vi "LidarTest.vi"() -> ()   [LabVIEW 2012]
uses:
  <instrlib>/Hokuyo URG Series/Public/Initialize-Standard.vi
  <instrlib>/Hokuyo URG Series/Hokuyo URG Series.lvlib
panel:
  out "Waveform Chart":i32(graph)
  out "size(s)":i32=961
  out "Direction":dbl[](array[numeric])
  out "Magnitude":dbl[](array[numeric])
  out "XY Graph":cluster{"X":dbl, "Y":dbl}[](graph)
  in  "polar attributes (hidden)":T1={"maximum"=30000.0, "minimum"=0.0, "clip to min"=FALSE, "log?(F)"=TRUE, "grid color"=6710886, "plot color"=65280, "fmt and prec"={"format"=enum."Decimal", "precision"=0}, "visible section"=8} {"minimum" format="%0.2f"; "maximum" format="%0.2f"}
  in  "Protocol":u32(ring)=2 items=["Convert to Latest", "SCIP 1.1", "SCIP 2.0"]
  in  "ID Query?":bool=TRUE
  in  "Checksum":bool
  in  "VISA resource name":refnum<visa-resource-name>="TCPIP::192.168.0.10::10940::SOCKET"
  in  "Stop":bool
  out "Data Aquired":picture
  in  "Grid Color":u32(colorbox)=16777222
  in  "Plot Color":u32(colorbox)=6618880
  in  "Max (m)":dbl=4.1
  in  "End Point":dbl=120.0
  in  "Start Point":dbl=-120.0
  in  "Cluster Count":dbl=1.0
  in  "Encoding Width":u16(ring)=3 items=["2 Byte"=2, "3 Byte"=3]
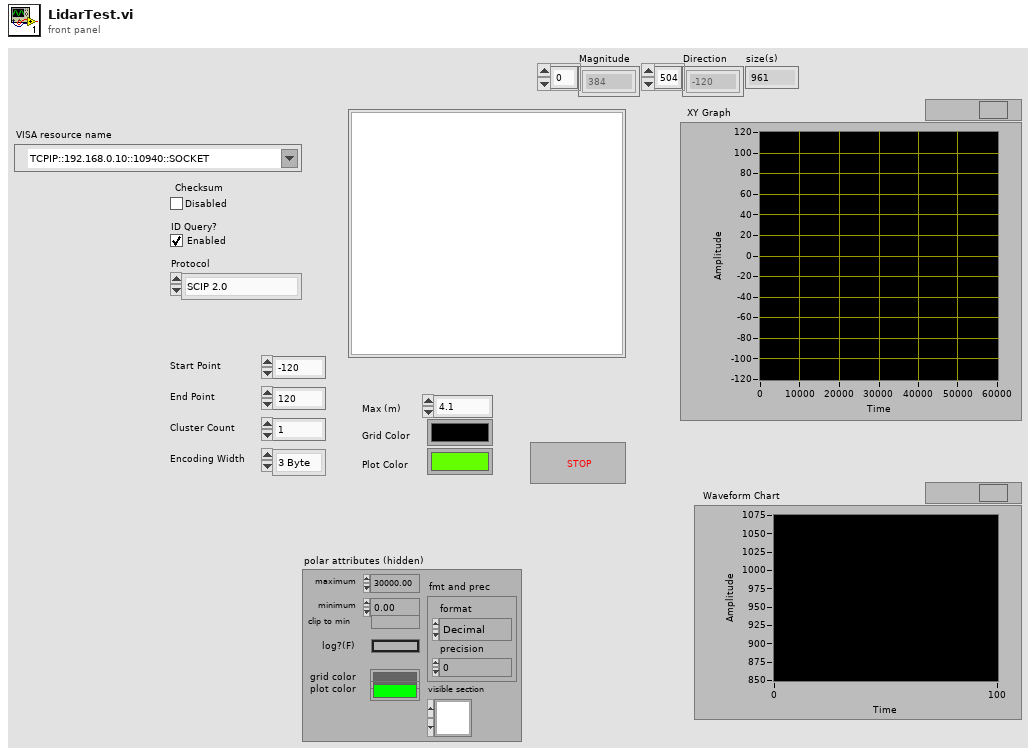
[diagram p1: front panel]
types:
  T1 = cluster{"maximum":dbl, "minimum":dbl, "clip to min":bool, "log?(F)":bool, "grid color":u32, "plot color":u32, "fmt and prec":cluster{"format":enum8{"Decimal", "Scientific", "Engineering", "Binary", "Octal", "Hex"}, "precision":u8}, "visible section":u16}
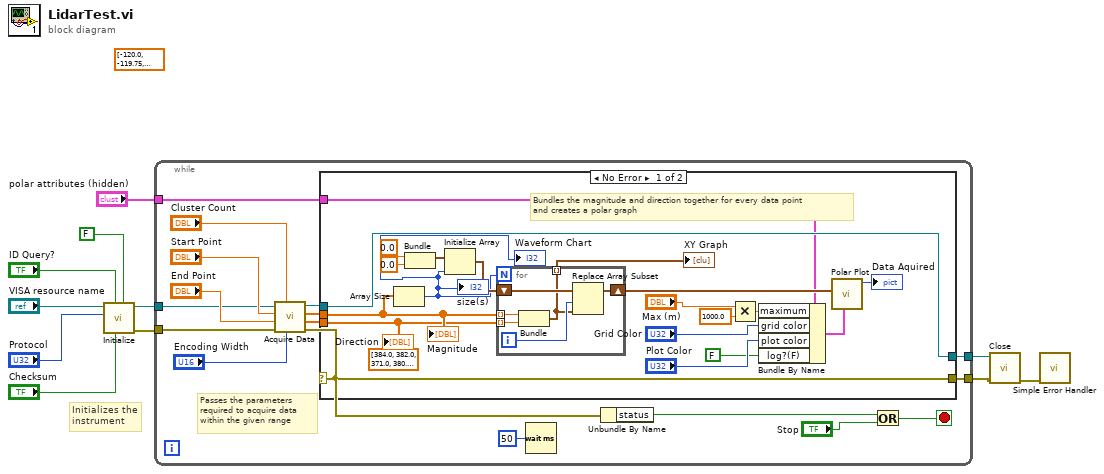
[diagram p0: block diagram]
diagram:
  (unwired) dbl[] [-120.0, -119.75, -119.5, -119.25, -119.0, -118.75, -118.5, -118.25, -118.0, -117.75, -117.5, -117.25, -117.0, -116.75, -116.5, -116.25, -116.0, -115.75, -115.5, -115.25, -115.0, -114.75, -114.5, -114.25, -114.0, -113.75, -113.5, -113.25, -113.0, -112.75, -112.5, -112.25, -112.0, -111.75, -111.5, -111.25, -111.0, -110.75, -110.5, -110.25, -110.0, -109.75, -109.5, -109.25, -109.0, -108.75, -108.5, -108.25, -108.0, -107.75, -107.5, -107.25, -107.0, -106.75, -106.5, -106.25, -106.0, -105.75, -105.5, -105.25, -105.0, -104.75, -104.5, -104.25, -104.0, -103.75, -103.5, -103.25, -103.0, -102.75, -102.5, -102.25, -102.0, -101.75, -101.5, -101.25, -101.0, -100.75, -100.5, -100.25, -100.0, -99.75, -99.5, -99.25, -99.0, -98.75, -98.5, -98.25, -98.0, -97.75, -97.5, -97.25, -97.0, -96.75, -96.5, -96.25, -96.0, -95.75, -95.5, -95.25, -95.0, -94.75, -94.5, -94.25, -94.0, -93.75, -93.5, -93.25, -93.0, -92.75, -92.5, -92.25, -92.0, -91.75, -91.5, -91.25, -91.0, -90.75, -90.5, -90.25, -90.0, -89.75, -89.5, -89.25, -89.0, -88.75, -88.5, -88.25, -88.0, -87.75, -87.5, -87.25, -87.0, -86.75, -86.5, -86.25, -86.0, -85.75, -85.5, -85.25, -85.0, -84.75, -84.5, -84.25, -84.0, -83.75, -83.5, -83.25, -83.0, -82.75, -82.5, -82.25, -82.0, -81.75, -81.5, -81.25, -81.0, -80.75, -80.5, -80.25, -80.0, -79.75, -79.5, -79.25, -79.0, -78.75, -78.5, -78.25, -78.0, -77.75, -77.5, -77.25, -77.0, -76.75, -76.5, -76.25, -76.0, -75.75, -75.5, -75.25, -75.0, -74.75, -74.5, -74.25, -74.0, -73.75, -73.5, -73.25, -73.0, -72.75, -72.5, -72.25, -72.0, -71.75, -71.5, -71.25, -71.0, -70.75, -70.5, -70.25, -70.0, -69.75, -69.5, -69.25, -69.0, -68.75, -68.5, -68.25, -68.0, -67.75, -67.5, -67.25, -67.0, -66.75, -66.5, -66.25, -66.0, -65.75, -65.5, -65.25, -65.0, -64.75, -64.5, -64.25, -64.0, -63.75, -63.5, -63.25, -63.0, -62.75, -62.5, -62.25, -62.0, -61.75, -61.5, -61.25, -61.0, -60.75, -60.5, -60.25, -60.0, -59.75, -59.5, -59.25, -59.0, -58.75, -58.5, -58.25, -58.0, -57.75, -57.5, -57.25, -57.0, -56.75, -56.5, -56.25, -56.0, -55.75, -55.5, -55.25, -55.0, -54.75, -54.5, -54.25, -54.0, -53.75, -53.5, -53.25, -53.0, -52.75, -52.5, -52.25, -52.0, -51.75, -51.5, -51.25, -51.0, -50.75, -50.5, -50.25, -50.0, -49.75, -49.5, -49.25, -49.0, -48.75, -48.5, -48.25, -48.0, -47.75, -47.5, -47.25, -47.0, -46.75, -46.5, -46.25, -46.0, -45.75, -45.5, -45.25, -45.0, -44.75, -44.5, -44.25, -44.0, -43.75, -43.5, -43.25, -43.0, -42.75, -42.5, -42.25, -42.0, -41.75, -41.5, -41.25, -41.0, -40.75, -40.5, -40.25, -40.0, -39.75, -39.5, -39.25, -39.0, -38.75, -38.5, -38.25, -38.0, -37.75, -37.5, -37.25, -37.0, -36.75, -36.5, -36.25, -36.0, -35.75, -35.5, -35.25, -35.0, -34.75, -34.5, -34.25, -34.0, -33.75, -33.5, -33.25, -33.0, -32.75, -32.5, -32.25, -32.0, -31.75, -31.5, -31.25, -31.0, -30.75, -30.5, -30.25, -30.0, -29.75, -29.5, -29.25, -29.0, -28.75, -28.5, -28.25, -28.0, -27.75, -27.5, -27.25, -27.0, -26.75, -26.5, -26.25, -26.0, -25.75, -25.5, -25.25, -25.0, -24.75, -24.5, -24.25, -24.0, -23.75, -23.5, -23.25, -23.0, -22.75, -22.5, -22.25, -22.0, -21.75, -21.5, -21.25, -21.0, -20.75, -20.5, -20.25, -20.0, -19.75, -19.5, -19.25, -19.0, -18.75, -18.5, -18.25, -18.0, -17.75, -17.5, -17.25, -17.0, -16.75, -16.5, -16.25, -16.0, -15.75, -15.5, -15.25, -15.0, -14.75, -14.5, -14.25, -14.0, -13.75, -13.5, -13.25, -13.0, -12.75, -12.5, -12.25, -12.0, -11.75, -11.5, -11.25, -11.0, -10.75, -10.5, -10.25, -10.0, -9.75, -9.5, -9.25, -9.0, -8.75, -8.5, -8.25, -8.0, -7.75, -7.5, -7.25, -7.0, -6.75, -6.5, -6.25, -6.0, -5.75, -5.5, -5.25, -5.0, -4.75, -4.5, -4.25, -4.0, -3.75, -3.5, -3.25, -3.0, -2.75, -2.5, -2.25, -2.0, -1.75, -1.5, -1.25, -1.0, -0.75, -0.5, -0.25, 0.0, 0.25, 0.5, 0.75, 1.0, 1.25, 1.5, 1.75, 2.0, 2.25, 2.5, 2.75, 3.0, 3.25, 3.5, 3.75, 4.0, 4.25, 4.5, 4.75, 5.0, 5.25, 5.5, 5.75, 6.0, 6.25, 6.5, 6.75, 7.0, 7.25, 7.5, 7.75, 8.0, 8.25, 8.5, 8.75, 9.0, 9.25, 9.5, 9.75, 10.0, 10.25, 10.5, 10.75, 11.0, 11.25, 11.5, 11.75, 12.0, 12.25, 12.5, 12.75, 13.0, 13.25, 13.5, 13.75, 14.0, 14.25, 14.5, 14.75, 15.0, 15.25, 15.5, 15.75, 16.0, 16.25, 16.5, 16.75, 17.0, 17.25, 17.5, 17.75, 18.0, 18.25, 18.5, 18.75, 19.0, 19.25, 19.5, 19.75, 20.0, 20.25, 20.5, 20.75, 21.0, 21.25, 21.5, 21.75, 22.0, 22.25, 22.5, 22.75, 23.0, 23.25, 23.5, 23.75, 24.0, 24.25, 24.5, 24.75, 25.0, 25.25, 25.5, 25.75, 26.0, 26.25, 26.5, 26.75, 27.0, 27.25, 27.5, 27.75, 28.0, 28.25, 28.5, 28.75, 29.0, 29.25, 29.5, 29.75, 30.0, 30.25, 30.5, 30.75, 31.0, 31.25, 31.5, 31.75, 32.0, 32.25, 32.5, 32.75, 33.0, 33.25, 33.5, 33.75, 34.0, 34.25, 34.5, 34.75, 35.0, 35.25, 35.5, 35.75, 36.0, 36.25, 36.5, 36.75, 37.0, 37.25, 37.5, 37.75, 38.0, 38.25, 38.5, 38.75, 39.0, 39.25, 39.5, 39.75, 40.0, 40.25, 40.5, 40.75, 41.0, 41.25, 41.5, 41.75, 42.0, 42.25, 42.5, 42.75, 43.0, 43.25, 43.5, 43.75, 44.0, 44.25, 44.5, 44.75, 45.0, 45.25, 45.5, 45.75, 46.0, 46.25, 46.5, 46.75, 47.0, 47.25, 47.5, 47.75, 48.0, 48.25, 48.5, 48.75, 49.0, 49.25, 49.5, 49.75, 50.0, 50.25, 50.5, 50.75, 51.0, 51.25, 51.5, 51.75, 52.0, 52.25, 52.5, 52.75, 53.0, 53.25, 53.5, 53.75, 54.0, 54.25, 54.5, 54.75, 55.0, 55.25, 55.5, 55.75, 56.0, 56.25, 56.5, 56.75, 57.0, 57.25, 57.5, 57.75, 58.0, 58.25, 58.5, 58.75, 59.0, 59.25, 59.5, 59.75, 60.0, 60.25, 60.5, 60.75, 61.0, 61.25, 61.5, 61.75, 62.0, 62.25, 62.5, 62.75, 63.0, 63.25, 63.5, 63.75, 64.0, 64.25, 64.5, 64.75, 65.0, 65.25, 65.5, 65.75, 66.0, 66.25, 66.5, 66.75, 67.0, 67.25, 67.5, 67.75, 68.0, 68.25, 68.5, 68.75, 69.0, 69.25, 69.5, 69.75, 70.0, 70.25, 70.5, 70.75, 71.0, 71.25, 71.5, 71.75, 72.0, 72.25, 72.5, 72.75, 73.0, 73.25, 73.5, 73.75, 74.0, 74.25, 74.5, 74.75, 75.0, 75.25, 75.5, 75.75, 76.0, 76.25, 76.5, 76.75, 77.0, 77.25, 77.5, 77.75, 78.0, 78.25, 78.5, 78.75, 79.0, 79.25, 79.5, 79.75, 80.0, 80.25, 80.5, 80.75, 81.0, 81.25, 81.5, 81.75, 82.0, 82.25, 82.5, 82.75, 83.0, 83.25, 83.5, 83.75, 84.0, 84.25, 84.5, 84.75, 85.0, 85.25, 85.5, 85.75, 86.0, 86.25, 86.5, 86.75, 87.0, 87.25, 87.5, 87.75, 88.0, 88.25, 88.5, 88.75, 89.0, 89.25, 89.5, 89.75, 90.0, 90.25, 90.5, 90.75, 91.0, 91.25, 91.5, 91.75, 92.0, 92.25, 92.5, 92.75, 93.0, 93.25, 93.5, 93.75, 94.0, 94.25, 94.5, 94.75, 95.0, 95.25, 95.5, 95.75, 96.0, 96.25, 96.5, 96.75, 97.0, 97.25, 97.5, 97.75, 98.0, 98.25, 98.5, 98.75, 99.0, 99.25, 99.5, 99.75, 100.0, 100.25, 100.5, 100.75, 101.0, 101.25, 101.5, 101.75, 102.0, 102.25, 102.5, 102.75, 103.0, 103.25, 103.5, 103.75, 104.0, 104.25, 104.5, 104.75, 105.0, 105.25, 105.5, 105.75, 106.0, 106.25, 106.5, 106.75, 107.0, 107.25, 107.5, 107.75, 108.0, 108.25, 108.5, 108.75, 109.0, 109.25, 109.5, 109.75, 110.0, 110.25, 110.5, 110.75, 111.0, 111.25, 111.5, 111.75, 112.0, 112.25, 112.5, 112.75, 113.0, 113.25, 113.5, 113.75, 114.0, 114.25, 114.5, 114.75, 115.0, 115.25, 115.5, 115.75, 116.0, 116.25, 116.5, 116.75, 117.0, 117.25, 117.5, 117.75, 118.0, 118.25, 118.5, 118.75, 119.0, 119.25, 119.5, 119.75, 120.0] ("Direction")
  # "Initializes the instrument"
  n1 = call-poly <instrlib>:"Initialize.vi"("Reset? (F: No)"=FALSE ("Reset Instrument (Disabled)"), "Checksum (Disabled)"="Checksum", "ID Query? (Enabled)"="ID Query?", "Protocol (2: SCIP 2.0)"="Protocol", "VISA resource name"="VISA resource name") -> ("error out"=w3:errorcluster, "VISA resource name out"=w4:refnum<visa-resource-name>)  [unwired: 5 in]
  n2 = while {
    tunnel: w4 -> [w16]
    tunnel: [w28] -> w11
    tunnel: [w27] -> w5
    tunnel: w3 -> [w15]
    tunnel: "polar attributes (hidden)" -> [w14]
    stop <- w24 stop-if-true
    # "Passes the parameters\nrequired to acquire data\nwithin the given range"
    n3 = call <instrlib>:"Acquire Data.vi"("Data Encoding Width (3 Byte)"="Encoding Width", "Cluster Count (1)"="Cluster Count", "error in (no error)"=w15, "End Point (120°)"="End Point", "Start Point (-120°)"="Start Point", "VISA resource name"=w16) -> ("error out"=w20:errorcluster, "Direction"=w21:dbl[], "Magnitude"=w22:dbl[], "VISA resource name out"=w23:refnum<visa-resource-name>)  [unwired: 2 in]
    n4 = case shown="No Error" w20 {
      selector: w20 -> [w46 w56]
      tunnel: [w46 w56] -> w28
      tunnel: w23 -> [w47 w55]
      tunnel: [w47 w55] -> w27
      tunnel: w22 -> [w41 _]
      tunnel: w21 -> [w40 _]
      tunnel: w14 -> [w37 _]
      frame No Error {
        (unwired) dbl[] [384.0, 382.0, 371.0, 380.0, 376.0, 360.0, 366.0, 379.0, 384.0, 369.0, 374.0, 371.0, 373.0, 374.0, 383.0, 390.0, 384.0, 366.0, 376.0, 374.0, 371.0, 381.0, 388.0, 385.0, 390.0, 381.0, 375.0, 373.0, 383.0, 388.0, 397.0, 393.0, 388.0, 390.0, 389.0, 389.0, 403.0, 404.0, 390.0, 402.0, 399.0, 393.0, 413.0, 426.0, 464.0, 531.0, 618.0, 493.0, 926.0, 958.0, 951.0, 943.0, 947.0, 943.0, 951.0, 932.0, 919.0, 930.0, 921.0, 929.0, 916.0, 921.0, 908.0, 896.0, 896.0, 896.0, 893.0, 891.0, 885.0, 878.0, 875.0, 852.0, 859.0, 861.0, 869.0, 859.0, 859.0, 846.0, 843.0, 835.0, 820.0, 845.0, 830.0, 836.0, 829.0, 834.0, 825.0, 815.0, 825.0, 822.0, 823.0, 828.0, 814.0, 807.0, 808.0, 801.0, 805.0, 797.0, 800.0, 791.0, 788.0, 784.0, 776.0, 782.0, 778.0, 788.0, 790.0, 769.0, 764.0, 761.0, 751.0, 769.0, 760.0, 758.0, 763.0, 762.0, 751.0, 745.0, 749.0, 746.0, 753.0, 746.0, 748.0, 743.0, 736.0, 728.0, 736.0, 731.0, 740.0, 733.0, 725.0, 725.0, 731.0, 718.0, 714.0, 730.0, 730.0, 727.0, 718.0, 718.0, 712.0, 704.0, 721.0, 723.0, 722.0, 713.0, 712.0, 701.0, 715.0, 711.0, 710.0, 701.0, 706.0, 712.0, 696.0, 688.0, 697.0, 697.0, 698.0, 703.0, 699.0, 684.0, 694.0, 692.0, 688.0, 696.0, 696.0, 696.0, 684.0, 680.0, 684.0, 676.0, 690.0, 682.0, 684.0, 683.0, 677.0, 662.0, 667.0, 677.0, 682.0, 680.0, 672.0, 671.0, 665.0, 649.0, 657.0, 664.0, 664.0, 659.0, 651.0, 655.0, 658.0, 645.0, 658.0, 653.0, 651.0, 652.0, 643.0, 640.0, 640.0, 644.0, 649.0, 645.0, 639.0, 650.0, 634.0, 634.0, 642.0, 632.0, 641.0, 648.0, 648.0, 642.0, 640.0, 623.0, 633.0, 615.0, 632.0, 630.0, 621.0, 624.0, 627.0, 617.0, 620.0, 626.0, 634.0, 627.0, 619.0, 623.0, 612.0, 616.0, 626.0, 628.0, 629.0, 621.0, 622.0, 624.0, 615.0, 618.0, 633.0, 627.0, 630.0, 616.0, 614.0, 618.0, 626.0, 625.0, 619.0, 622.0, 624.0, 613.0, 613.0, 610.0, 613.0, 619.0, 614.0, 605.0, 616.0, 612.0, 616.0, 610.0, 626.0, 633.0, 624.0, 628.0, 636.0, 627.0, 615.0, 628.0, 630.0, 636.0, 646.0, 644.0, 643.0, 644.0, 643.0, 642.0, 645.0, 649.0, 647.0, 655.0, 656.0, 656.0, 662.0, 671.0, 671.0, 677.0, 682.0, 714.0, 782.0, 698.0, 656.0, 1796.0, 1785.0, 1801.0, 1795.0, 1790.0, 1793.0, 1793.0, 1789.0, 1808.0, 1803.0, 1799.0, 954.0, 1039.0, 943.0, 925.0, 924.0, 933.0, 927.0, 911.0, 913.0, 904.0, 920.0, 912.0, 862.0, 866.0, 852.0, 833.0, 806.0, 806.0, 828.0, 833.0, 812.0, 812.0, 799.0, 795.0, 808.0, 802.0, 806.0, 798.0, 791.0, 801.0, 796.0, 796.0, 805.0, 803.0, 814.0, 812.0, 827.0, 816.0, 830.0, 833.0, 838.0, 822.0, 828.0, 823.0, 826.0, 820.0, 812.0, 813.0, 807.0, 804.0, 816.0, 810.0, 802.0, 802.0, 797.0, 809.0, 856.0, 971.0, 962.0, 953.0, 928.0, 916.0, 907.0, 890.0, 881.0, 880.0, 866.0, 870.0, 976.0, 1046.0, 1010.0, 1805.0, 1794.0, 1794.0, 1665.0, 1451.0, 1411.0, 1415.0, 1442.0, 1429.0, 1454.0, 1453.0, 1437.0, 1427.0, 1385.0, 1346.0, 1314.0, 1245.0, 1139.0, 1131.0, 1118.0, 1125.0, 1115.0, 1120.0, 1120.0, 1139.0, 1141.0, 1147.0, 1155.0, 1167.0, 1176.0, 1187.0, 1199.0, 1214.0, 1229.0, 1263.0, 1263.0, 1279.0, 1304.0, 1328.0, 1321.0, 1311.0, 1326.0, 1317.0, 1316.0, 1301.0, 1278.0, 1277.0, 1295.0, 1253.0, 1256.0, 1270.0, 1268.0, 1256.0, 1268.0, 1271.0, 1231.0, 1259.0, 1220.0, 1229.0, 1229.0, 1264.0, 1234.0, 1226.0, 60000.0, 1243.0, 1249.0, 1275.0, 2345.0, 1307.0, 1358.0, 1316.0, 1304.0, 1304.0, 1244.0, 1174.0, 1183.0, 1220.0, 1241.0, 1234.0, 1231.0, 1232.0, 1227.0, 1231.0, 1269.0, 1360.0, 1285.0, 2288.0, 2298.0, 2316.0, 2335.0, 2353.0, 2377.0, 2389.0, 2410.0, 2423.0, 2444.0, 2464.0, 2483.0, 2504.0, 2529.0, 2529.0, 2544.0, 2562.0, 2559.0, 2565.0, 2558.0, 2565.0, 2568.0, 2550.0, 2531.0, 2494.0, 2465.0, 2470.0, 1035.0, 1042.0, 1031.0, 1030.0, 1025.0, 1019.0, 1032.0, 1024.0, 1008.0, 1026.0, 1034.0, 993.0, 1002.0, 994.0, 1007.0, 1020.0, 1032.0, 1039.0, 1040.0, 1038.0, 1093.0, 2627.0, 2611.0, 2605.0, 2604.0, 2598.0, 2602.0, 2599.0, 2598.0, 2590.0, 2598.0, 2576.0, 2577.0, 2570.0, 2557.0, 2557.0, 2554.0, 2553.0, 2549.0, 2536.0, 2531.0, 2524.0, 2516.0, 2532.0, 2518.0, 993.0, 999.0, 973.0, 989.0, 983.0, 2493.0, 2501.0, 2497.0, 2488.0, 2491.0, 2480.0, 2473.0, 2477.0, 2470.0, 2474.0, 2472.0, 2474.0, 2455.0, 2458.0, 2455.0, 2455.0, 2460.0, 2450.0, 2455.0, 2447.0, 2442.0, 2445.0, 2443.0, 2440.0, 759.0, 760.0, 742.0, 743.0, 738.0, 729.0, 727.0, 732.0, 735.0, 732.0, 722.0, 719.0, 729.0, 729.0, 722.0, 725.0, 734.0, 724.0, 725.0, 722.0, 732.0, 726.0, 737.0, 759.0, 741.0, 772.0, 850.0, 910.0, 2175.0, 2176.0, 2118.0, 1875.0, 1834.0, 1815.0, 1871.0, 1932.0, 2018.0, 2087.0, 2106.0, 2083.0, 1971.0, 1947.0, 1934.0, 1919.0, 1928.0, 1914.0, 1916.0, 1917.0, 1897.0, 1907.0, 1909.0, 1902.0, 1899.0, 1904.0, 1907.0, 1897.0, 1899.0, 1892.0, 1888.0, 1895.0, 1897.0, 1902.0, 1900.0, 1875.0, 1894.0, 1889.0, 1889.0, 1888.0, 1890.0, 1879.0, 1883.0, 1875.0, 1879.0, 1881.0, 1887.0, 1878.0, 1873.0, 1880.0, 1874.0, 1868.0, 1873.0, 1877.0, 1869.0, 1880.0, 1882.0, 1869.0, 1827.0, 1508.0, 1291.0, 1187.0, 1175.0, 1187.0, 1178.0, 1165.0, 1172.0, 1168.0, 1189.0, 1210.0, 1201.0, 1183.0, 1189.0, 1207.0, 1190.0, 1173.0, 1179.0, 1195.0, 1208.0, 1214.0, 1203.0, 1203.0, 1209.0, 1216.0, 1219.0, 1216.0, 1210.0, 1195.0, 1182.0, 1182.0, 1185.0, 1181.0, 1185.0, 1188.0, 1182.0, 1185.0, 1177.0, 1193.0, 1213.0, 1331.0, 1526.0, 1573.0, 1579.0, 1589.0, 1586.0, 1586.0, 1585.0, 1602.0, 1591.0, 1585.0, 1601.0, 1639.0, 1938.0, 1915.0, 1916.0, 1915.0, 1891.0, 1887.0, 1877.0, 1854.0, 1839.0, 1825.0, 1805.0, 1805.0, 1799.0, 1819.0, 1984.0, 2281.0, 2266.0, 2250.0, 2242.0, 2233.0, 2213.0, 2192.0, 2181.0, 2177.0, 2151.0, 2166.0, 2237.0, 2371.0, 2756.0, 2764.0, 2725.0, 2738.0, 2773.0, 2802.0, 2821.0, 2834.0, 2827.0, 2829.0, 2809.0, 2800.0, 2788.0, 2753.0, 2652.0, 2618.0, 1670.0, 1566.0, 1564.0, 1565.0, 1550.0, 1554.0, 1551.0, 1544.0, 1551.0, 1545.0, 1551.0, 1566.0, 1585.0, 1563.0, 2399.0, 2385.0, 2395.0, 2381.0, 2380.0, 2365.0, 2341.0, 2339.0, 2317.0, 2305.0, 2303.0, 2292.0, 2287.0, 2279.0, 2269.0, 2241.0, 2207.0, 1832.0, 1723.0, 1644.0, 1579.0, 1525.0, 1491.0, 1484.0, 1480.0, 1475.0, 1471.0, 1478.0, 1471.0, 1465.0, 1458.0, 1449.0, 1451.0, 1456.0, 1459.0, 1465.0, 1468.0, 1470.0, 1462.0, 1465.0, 1481.0, 1508.0, 1540.0, 1713.0, 1650.0, 1653.0, 1630.0, 1629.0, 1549.0, 1537.0, 1535.0, 1561.0, 1647.0, 1684.0, 2021.0, 2050.0, 2044.0, 2048.0, 2040.0, 2020.0, 2005.0, 1990.0, 1770.0, 1745.0, 1750.0, 1756.0, 1801.0, 1962.0, 1966.0, 1975.0, 1978.0, 1966.0, 1967.0, 1953.0, 1950.0, 1944.0, 1937.0, 1941.0, 1940.0, 1938.0, 1928.0, 1926.0, 1918.0, 1905.0, 1912.0, 1901.0, 1905.0, 1898.0, 1889.0, 1889.0, 1884.0, 1882.0, 1869.0, 1880.0, 1879.0, 1867.0, 1864.0, 1858.0, 1852.0, 1837.0, 1845.0, 1845.0, 1848.0, 1839.0, 1832.0, 1832.0, 1833.0, 1834.0, 1829.0, 1827.0, 1812.0, 1812.0, 1813.0, 1804.0, 1809.0, 1807.0, 1812.0, 1797.0, 1795.0, 1791.0, 1782.0, 1783.0, 1791.0, 1792.0, 1789.0, 1748.0, 1668.0, 1676.0, 1669.0, 1668.0, 1661.0, 1675.0, 1661.0, 1656.0, 1659.0, 1648.0, 1644.0, 1658.0, 1652.0, 1634.0, 1639.0, 1632.0, 1637.0, 1632.0, 1626.0, 1616.0, 1486.0, 1188.0, 1110.0, 1084.0, 1086.0, 1090.0, 1094.0, 1094.0, 1096.0, 1104.0, 1090.0, 1092.0, 1086.0, 1088.0, 1089.0, 1080.0, 1090.0, 1086.0, 1087.0, 1075.0, 1075.0, 1081.0, 1087.0, 1082.0, 1067.0, 1069.0, 1072.0, 1071.0, 1087.0, 1094.0, 1112.0, 1116.0, 1124.0, 1149.0, 1233.0, 1234.0, 1232.0, 1233.0, 1234.0, 1226.0, 1226.0, 1220.0, 1225.0, 1234.0, 1252.0, 1435.0, 1228.0, 1653.0, 1330.0, 1664.0, 1676.0, 1670.0, 1679.0, 1433.0, 1202.0] ("Magnitude")
        # "Bundles the magnitude and direction together for every data point\nand creates a polar graph"
        n5 = Array Size(array=w41) -> (size(s)=w29:i32)
        "size(s)" <- w29
        "Waveform Chart" <- w29
        n6 = Bundle(0.0, 0.0) -> (w43:cluster{dbl, dbl})  [unwired: 1 in]
        n7 = Initialize Array(w43, w29) -> (w42:cluster{dbl, dbl}[])
        n8 = for {
          N: w29 -> [_]
          shift-right: [w50] -> w39
          shift-left: w42 -> [w51]
          tunnel: w41 -> [w54] mode=indexing
          tunnel: w40 -> [w53] mode=indexing
          tunnel: [w49] -> w30 mode=indexing
          i -> [w52]
          n9 = Bundle(w54, w53) -> (w49:cluster{dbl, dbl})  [unwired: 1 in]
          n10 = Replace Array Subset(array=w51, new element=w49, index=w52) -> (w50:cluster{dbl, dbl}[])
        }
        "XY Graph" <- w30
        n11 = Multiply(x="Max (m)", y=1000.0) -> (x*y=w33:dbl)
        n12 = Bundle By Name(cluster=w37, "maximum"=w33, "grid color"="Grid Color", "plot color"="Plot Color", "log?(F)"=FALSE) -> (w38:T1)
        n13 = call <vilib>:"Polar Plot.vi"("polar attributes"=w38, "data array [mag, phase (deg)]"=w39) -> ("new picture"=→"Data Aquired":picture)  [unwired: 9 in]
        "Magnitude" <- w41
        "Direction" <- w40
      }
      frame Error {
      }
    }
    n14 = Wait (ms)(milliseconds to wait=u32 50) -> ()  [unwired: 1 out]
    n15 = Unbundle By Name(w20) -> ("status"=w26:bool)
    n16 = Or(x=w26, y="Stop") -> (x .or. y?=w24:bool)
  }
  n17 = call <instrlib>:"Close.vi"("error in (no error)"=w11, "VISA resource name"=w5) -> ("error out"=w9:errorcluster)  [unwired: 9 in]
  n18 = call <vilib>:"Simple Error Handler.vi"("error in (no error)"=w9) -> ()  [unwired: 4 in, 5 out]
